vi "Graph 2.vi"() -> ()   [LabVIEW 2024]
panel:
  out "XY Graph":cluster{"X":dbl, "Y":dbl}[](graph)
  out "Waveform Chart 2":cluster{dbl, dbl}(graph)
  in  "stop 2":bool
  in  "stop":bool
  out "Waveform Chart":cluster{dbl, dbl}(graph)
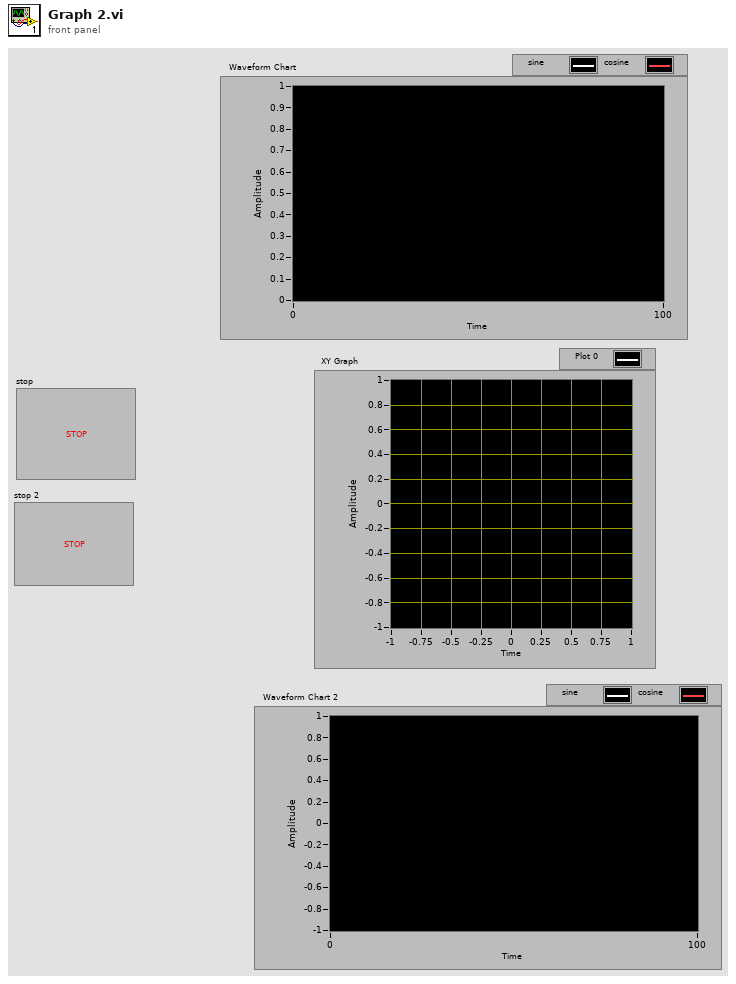
[diagram p1: front panel]
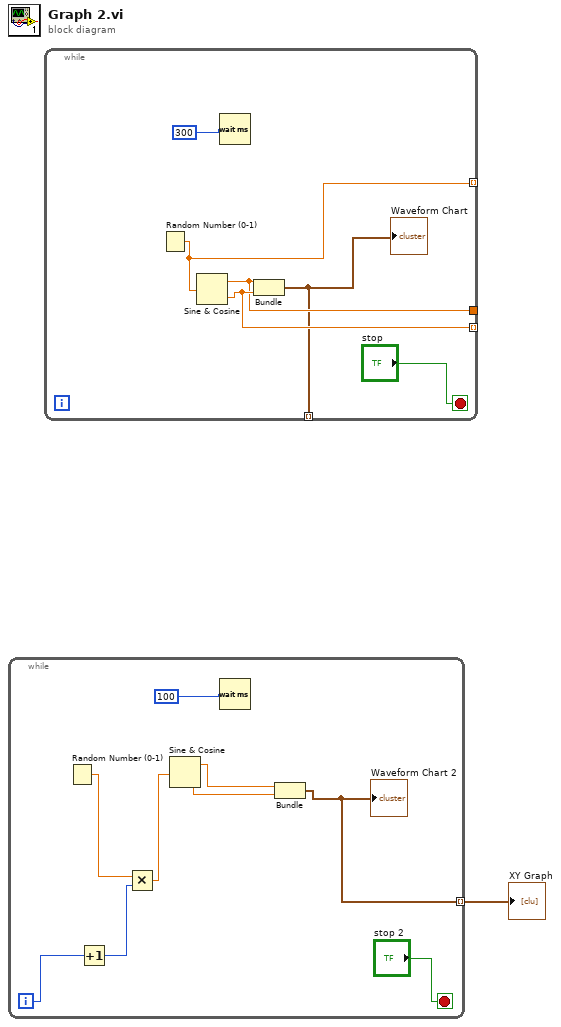
[diagram p0: block diagram]
diagram:
  n1 = while {
    tunnel: [w2] -> w1 mode=indexing
    i -> [w6]
    stop <- "stop 2" stop-if-true
    n2 = Random Number (0-1)() -> (number: 0 to 1=w5:dbl)
    n3 = Increment(x=w6) -> (x+1=w4:i32)
    n4 = Multiply(x=w5, y=w4) -> (x*y=w3:dbl)
    n5 = Sine & Cosine(0:w3) -> (1:w8:dbl, 2:w7:dbl)
    n6 = Wait (ms)(milliseconds to wait=u32 100) -> ()  [unwired: 1 out]
    n7 = Bundle(w8, w7) -> (w2:cluster{dbl, dbl})  [unwired: 1 in]
    "Waveform Chart 2" <- w2
  }
  "XY Graph" <- w1
  n8 = while {
    tunnel: [w14] -> _ mode=indexing
    tunnel: [w13] -> _
    tunnel: [w12] -> _ mode=indexing
    tunnel: [w11] -> _ mode=indexing
    stop <- "stop" stop-if-true
    n9 = Random Number (0-1)() -> (number: 0 to 1=w12:dbl)
    n10 = Sine & Cosine(0:w12) -> (1:w13:dbl, 2:w14:dbl)
    n11 = Wait (ms)(milliseconds to wait=u32 300) -> ()  [unwired: 1 out]
    n12 = Bundle(w13, w14) -> (w11:cluster{dbl, dbl})  [unwired: 1 in]
    "Waveform Chart" <- w11
  }
